vi "Write Activate Microgrid Msg.vi"(10 "Activate Microgrid Msg":refnum<class "Activate Microgrid Msg.lvclass">, 11 "Remote Operation Abstract in":refnum<class "Remote Operation Abstract.lvclass">) -> (3 "Remote Operation Abstract out":refnum<class "Remote Operation Abstract.lvclass">)   [LabVIEW 2018, in "Remote Operation Abstract.lvlib" / "Remote Operation Abstract.lvclass"]
uses:
  Remote Operation Abstract.lvclass
  Remote Operation Abstract Messages/Activate Microgrid Msg/Activate Microgrid Msg.lvclass
  Remote Operation Abstract.lvclass/Remote Operation Abstract.ctl
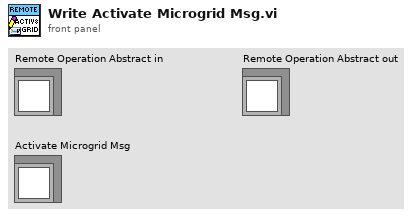
[diagram p1: front panel]
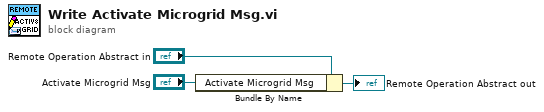
[diagram p0: block diagram]
diagram:
  n1 = Bundle By Name(cluster="Remote Operation Abstract in", "Activate Microgrid Msg"="Activate Microgrid Msg") -> (→"Remote Operation Abstract out":refnum<class "Remote Operation Abstract.lvclass">)
